vi "HexDAQ.vi"() -> ()   [LabVIEW 2016]
uses:
  input_params.ctl
  refs_front_panel.ctl
  <extravilib>/ChannelInstances/Tag-a[.](c(a[.](stamp),a[.](dbl)))/Read With Abort.vi
  <extravilib>/ChannelInstances/Tag-bool/Read With Abort.vi
  <extravilib>/ChannelInstances/Tag-t'Input_parameters.ctl'/Write With Abort.vi
  <extravilib>/ChannelInstances/Tag-str/Write With Abort.vi
  <extravilib>/ChannelInstances/Tag-bool/Write With Abort.vi
  <extravilib>/ChannelInstances/Tag-t'Input_parameters.ctl'/Instantiate.vi
  <extravilib>/ChannelInstances/Tag-str/Instantiate.vi
  <extravilib>/ChannelInstances/Tag-a[.](c(a[.](stamp),a[.](dbl)))/Instantiate.vi
  <extravilib>/ChannelInstances/Tag-t'Env_data.ctl'/Instantiate.vi
  <extravilib>/ChannelInstances/Tag-bool/Instantiate.vi
  <extravilib>/ChannelInstances/Tag-a[.](c(a[.](stamp),a[.](dbl)))/Endpoint.vi
  <extravilib>/ChannelInstances/Tag-bool/Endpoint.vi
  <extravilib>/ChannelInstances/Tag-t'Input_parameters.ctl'/Endpoint.vi
  <extravilib>/ChannelInstances/Tag-str/Endpoint.vi
  <extravilib>/ChannelInstances/Tag-bool.lvlib
  <extravilib>/ChannelInstances/Tag-a[.](c(a[.](stamp),a[.](dbl))).lvlib
  <extravilib>/ChannelInstances/Tag-str.lvlib
  <extravilib>/ChannelInstances/Tag-t'Input_parameters.ctl'.lvlib
  user32.dll
panel:
  in  "CV Switch Delay (s)":dbl
  in  "IV Switch Delay (s)":dbl
  in  "CV voltage file":path=path "C:/Users/Administrator/Desktop/HGCAL_sensor_tests/config/voltagesCV.txt"
  in  "IV voltage file":path=path "C:/Users/Administrator/Desktop/HGCAL_sensor_tests/config/voltagesIV.txt"
  in  "Abort 2":bool
  in  "Invert polarity":bool
  in  "No CV corrections":bool
  in  "Total curr/vlt \nevery x pads":i32=10
  in  "Disable Switchcard":bool
  in  "Comments (saved in data file)":string
  in  "Needle?":bool
  out "Total current":cluster{i32[], dbl[]}[](graph) caption="XY Graph"
  in  "CV voltage delay (s)":dbl=20.0
  in  "Sensor type":T1(ring)
  in  "Custom pad scan":string
  in  "Measurement type":T2(ring)=enum."Debug"
  in  "Hex pad numbers?":bool=TRUE
  in  "?":refnum<k7>(container)
  in  "Custom\nvoltages IV":string
  out "Single channel":cluster{"X array":dbl[], "Y array":dbl[]}[](graph) caption="XY Graph"
  in  "Repeat":i32=1
  in  "LCR signal voltage (V)":dbl=0.501
  in  "LCR signal frequenzy (kHz)":dbl=50.0 format="%#_13g"
  in  "Sampling number":i32=3
  in  "DMM device":T3(ring)=enum."Keithley6487"
  in  "Take environmental sensor data from":T4(ring)=enum."Switch Matrix"
  out "Environmental data":cluster{timestamp[], dbl[]}[](graph)
  out "Elapsed time":dbl format="%<%H:%M:%S>t"
  out "Estimated remaining time":dbl format="%<%H:%M:%S>t"
  out "Channel values":cluster{i32[], dbl[]}[](graph) caption="XY Graph"
  out "Current channel":dbl format="%#_13g"
  out "Current voltage (V)":dbl format="%#_13g"
  in  "Abort":bool
  in  "Output file":refnum<k7>(container) caption="Preview data file"
  in  "END DAQ":bool
  in  "START DAQ":bool
  in  "Custom\nvoltages CV":string
  in  "Data storage location (def: ./results)":path=path "C:/Users/Administrator/cernbox/HGCAL test results/Data"
  in  "Plot after execution?":bool=TRUE
  in  "Voltage limit (V)":dbl=1000.0
  in  "Compliance  level (uA)":dbl=500.0
  in  "VISA resource name LCR":refnum<visa-resource-name>="LCR_E4980"
  in  "VISA resource name DMM":refnum<visa-resource-name>="KEITHLEY_6487"
  in  "VISA resource name source":refnum<visa-resource-name>="Source_2410"
  in  "IV voltage delay (s)":dbl=5.0
  in  "Display/needle\nchannel":i32=144
  in  "Open after execution?":bool
  in  "Identifier (eg. wafer number)":string="Debug"
  # "HexDAQ\nThe LabVIEW program for HGCAL sensor tests\nFeedback and bug reports to andreas.alexander.maier@cern.ch"
  # "Measurement settings"
  # "Bookkeeping settings"
  # "VISA settings"
  # "Both are used to determine \nthe folder and file names"
  # "Device settings"
  # "Timing settings"
  # "Debug settings"
  # "Data processing settings"
  # "Ctrl+H for full display"
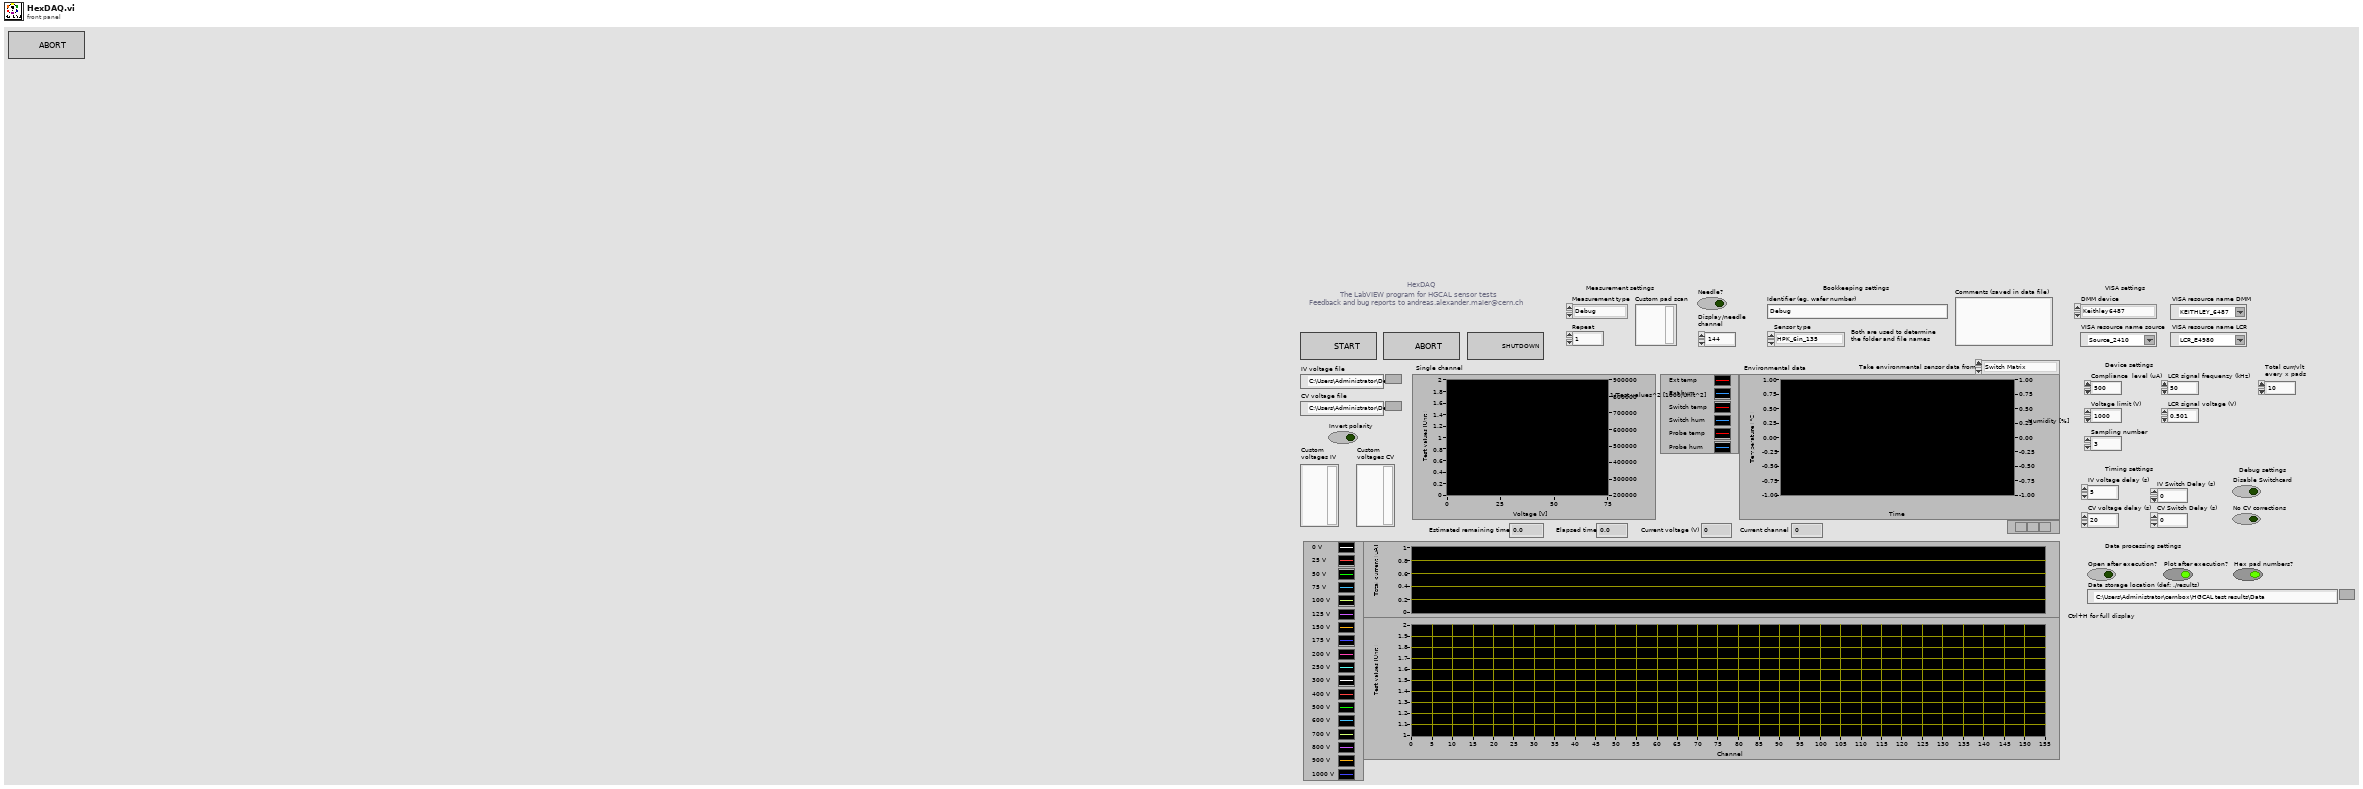
[diagram p1: front panel]
types:
  T1 = enum16{"HPK_6in_135", "HPK_8in_256", "IFX_8in_256", "Diode", "HPK_6in_256", "Full matrix"}
  T2 = enum16{"IV", "CV", "Debug", "Test_contact", "IV+CV"}
  T3 = enum16{"Keithley2001", "Keithley2450", "Keithley2410", "Keithley6487"}
  T4 = enum16{"Sensirion sht1x/7x", "Switch Matrix", "Probecard"}
  T5 = typedef "refs_front_panel.ctl" = cluster{"Current voltage (V)":refnum<vi>, "Elapsed time":refnum<vi>, "Current channel":refnum<vi>, "Abort":refnum<vi>, "Estimated remaining time":refnum<vi>, "Channel values XYGraph":refnum<vi>, "Single channel XYGraph":refnum<vi>, "Total current XYGraph":refnum<vi>}
  T6 = typedef "input_params.ctl" = cluster{"Measurement type":enum16{"IV", "CV", "Debug", "Test_contact"}, "Sensor type":enum16{"HPK_6in_135", "HPK_8in_256", "IFX_8in_256", "Diode", "HPK_6in_256", "Full matrix"}, "Identifier":string, "Open after execution?":bool, "Plot after execution?":bool, "Display channel":i32, "Voltage Delay (s)":dbl, "Switch Delay (s)":dbl, "VISA resource name source":refnum<visa-resource-name>, "VISA resource name DMM":refnum<visa-resource-name>, "VISA resource name LCR":refnum<visa-resource-name>, "Compliance  Level (A)":dbl, "Voltage Limit (V)":dbl, "Data storage location":string, "Scan voltages":string, "Use source as DMM?":bool, "LCR signal frequenzy (Hz)":dbl, "DMM device":enum16{"Keithley2001", "Keithley2450", "Keithley2410", "Keithley6487"}, "Sampling number":i32, "Use env. sensors on":enum16{"Sensirion sht1x/7x", "Switch Matrix", "Probecard"}, "Switchboard Handle":u32, "Use Switchboard":bool, "LCR signal voltage (V)":dbl, "Repeat":i32, "Scan voltages IV":string, "Scan voltages CV":string, "Hex pad numbers?":bool, "Set measurement type":enum16{"IV", "CV", "Debug", "Test_contact", "IV+CV"}, "Custom pad scan":string, "IV voltage Delay (s)":dbl, "CV voltage Delay (s)":dbl, "Needle measurement?":bool, "Comments":string, "LCR signal frequenzy (kHz)":dbl, "Compliance  Level (uA)":dbl, "Open Correction Array":dbl[][], "Current set voltage":dbl, "Last set voltage":dbl, "Current channel":i32, "Last OpenCorrection index":i32, "Total curr/vltg every x steps":i32, "Current channel iteration":i32, "No CV corrections":bool, "Mapfile":string, "Corrfile":string, "Invert polarity":bool, "IV voltage file":path, "CV voltage file":path, "IV Switch Delay (s)":dbl, "CV Switch Delay (s)":dbl}
  T7 = typedef "Tag-t'Input_parameters.ctl'.lvlib/))Channel.ctl" = refnum<queue>
  T8 = typedef "Tag-str.lvlib/))Channel.ctl" = refnum<queue>
  T9 = typedef "data_dynamic.ctl" = cluster{"Output file":path, "Y-label text":string, "Current set voltage":dbl, "Set voltage column":dbl[], "Pad number column":dbl[], "Data  column":dbl[], "Number of voltages":i32, "Compliance current (A)":dbl, "Geofile":string, "Peak voltage":dbl, "Hex PDF file":string, "Voltage array":dbl[], "Total current column":dbl[], "Timestamp column":dbl[], "Data name":string, "Data unit":string, "2nd data column":dbl[], "2nd data name":string, "2nd data unit":string, "3rd data column":dbl[], "4th data column":dbl[], "3rd data name":string, "3rd data unit":string, "4th data name":string, "4th data unit":string, "Actual voltage column":dbl[], "2nd Y-label text":string, "Single channel plot":path, "Temperature column":dbl[], "Humidity column":dbl[], "Channel switch array":i32[], "1st single plot name":string, "2nd single plot name":string, "All channels plot":path, "HexPlot command":string, "Custom channel array":i32[], "Data  error column":dbl[], "2nd data  error column":dbl[], "3rd data error column":dbl[], "4th data  error column":dbl[], "Total current plot":path, "5th data column":dbl[], "5th data  error column":dbl[], "6th data column":dbl[], "6th data  error column":dbl[], "5th data name":string, "5th data unit":string, "6th data name":string, "6th data unit":string, "HexPlot matrix command":string}
  T10 = typedef "Tag-bool.lvlib/))Channel.ctl" = refnum<queue>
  T11 = typedef "Tag-a[.](c(a[.](stamp),a[.](dbl))).lvlib/))Channel.ctl" = refnum<queue>
  T12 = typedef "Tag-t'Env_data.ctl'.lvlib/))Channel.ctl" = refnum<queue>
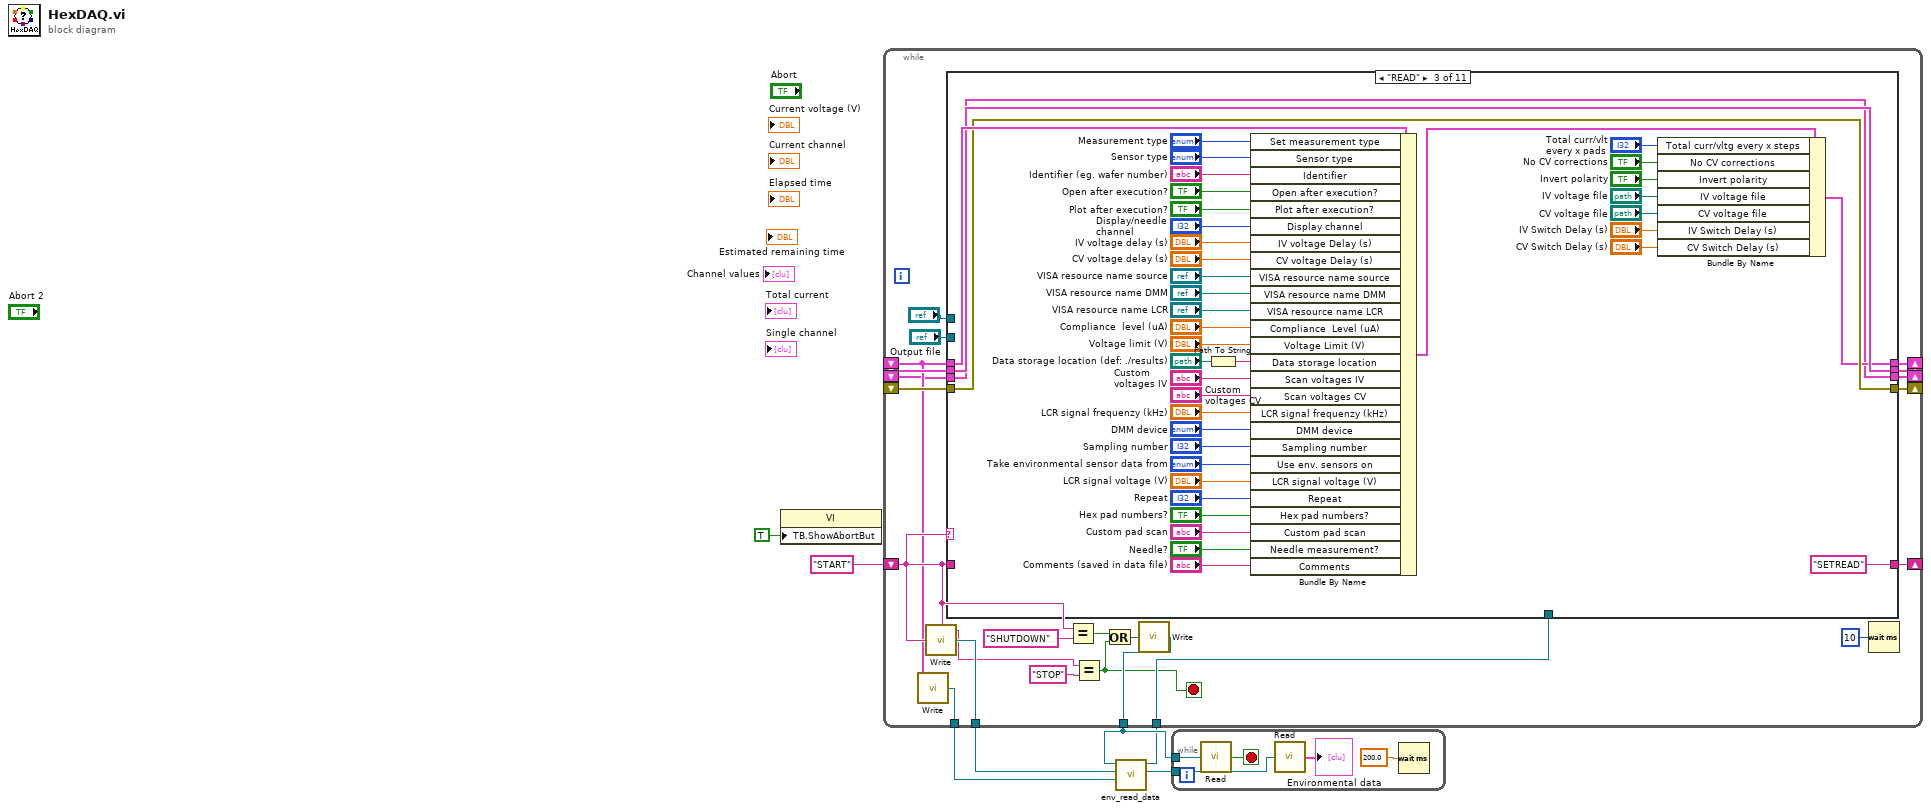
[diagram p0: block diagram]
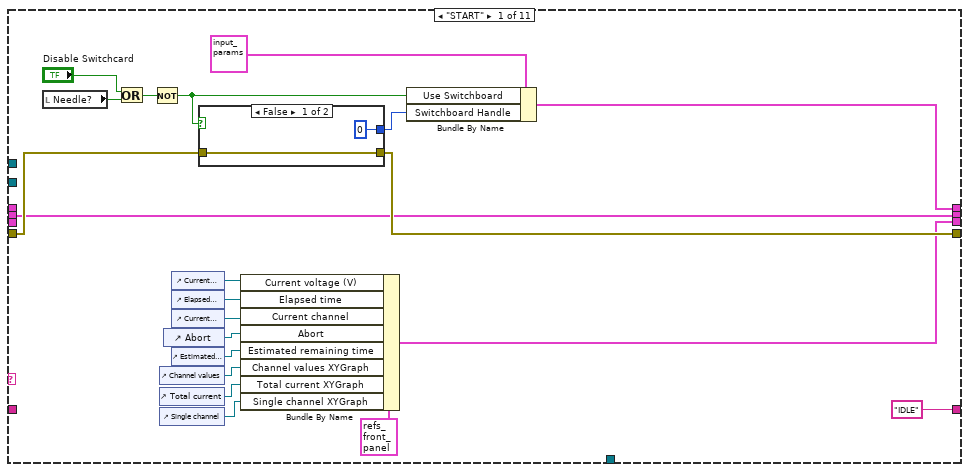
[diagram p2: hidden frame]
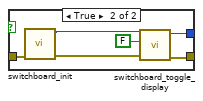
[diagram p3: hidden frame]
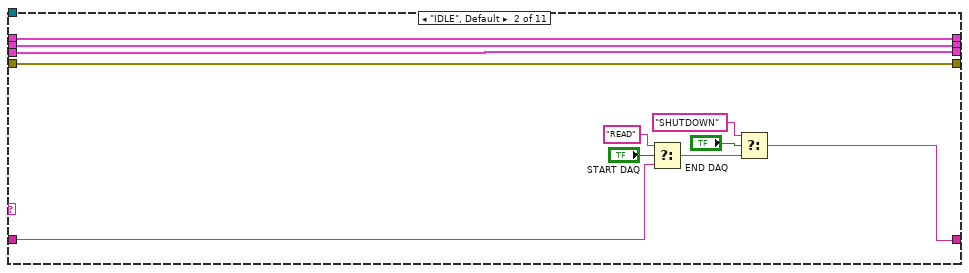
[diagram p4: hidden frame]
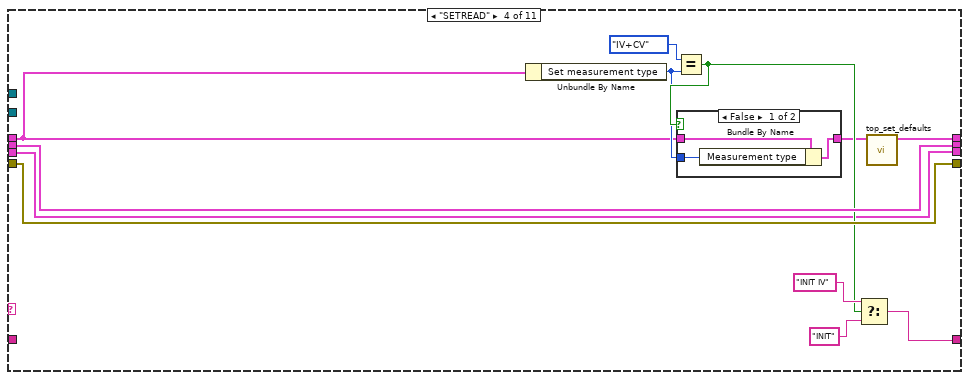
[diagram p5: hidden frame]
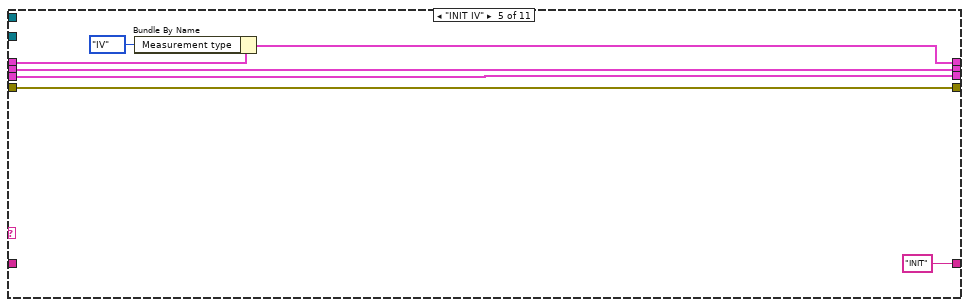
[diagram p7: hidden frame]
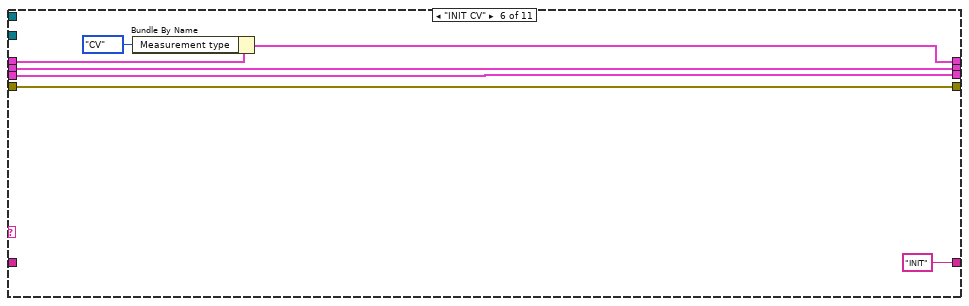
[diagram p8: hidden frame]
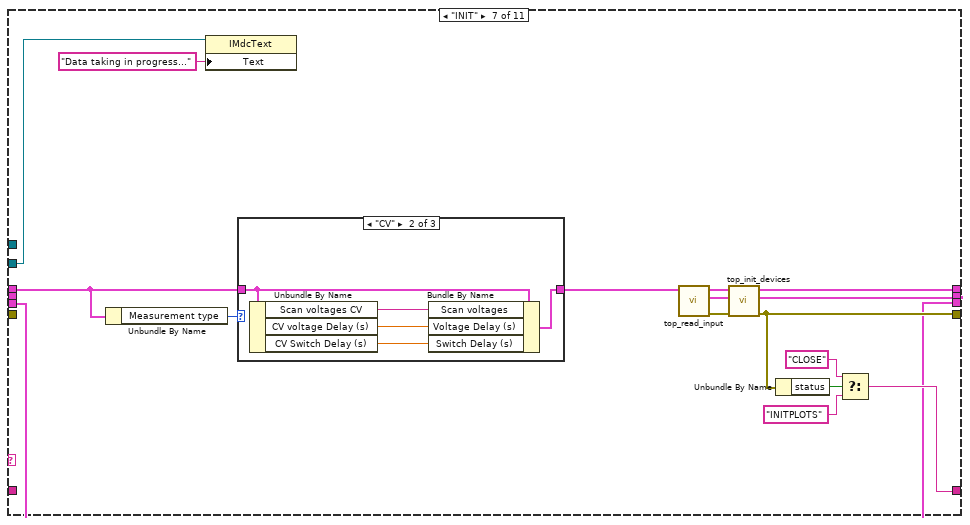
[diagram p9: hidden frame]
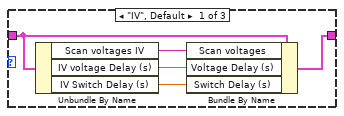
[diagram p10: hidden frame]
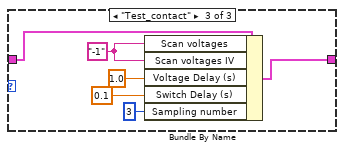
[diagram p11: hidden frame]
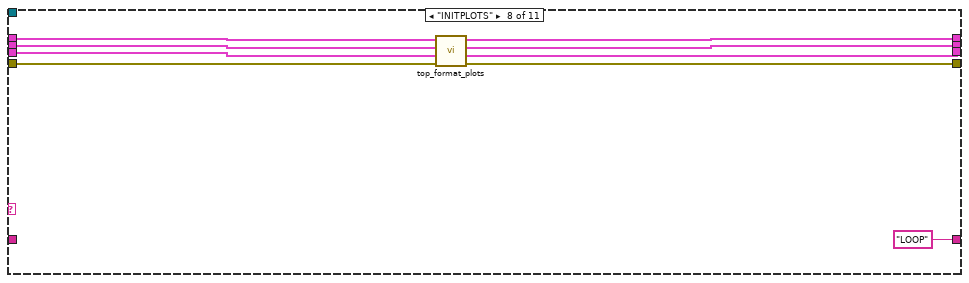
[diagram p12: hidden frame]
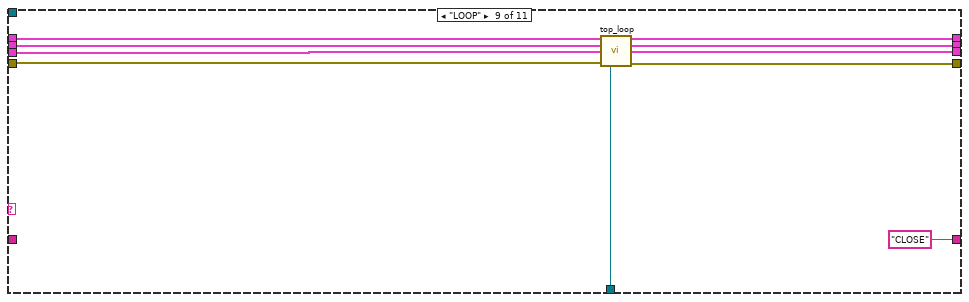
[diagram p13: hidden frame]
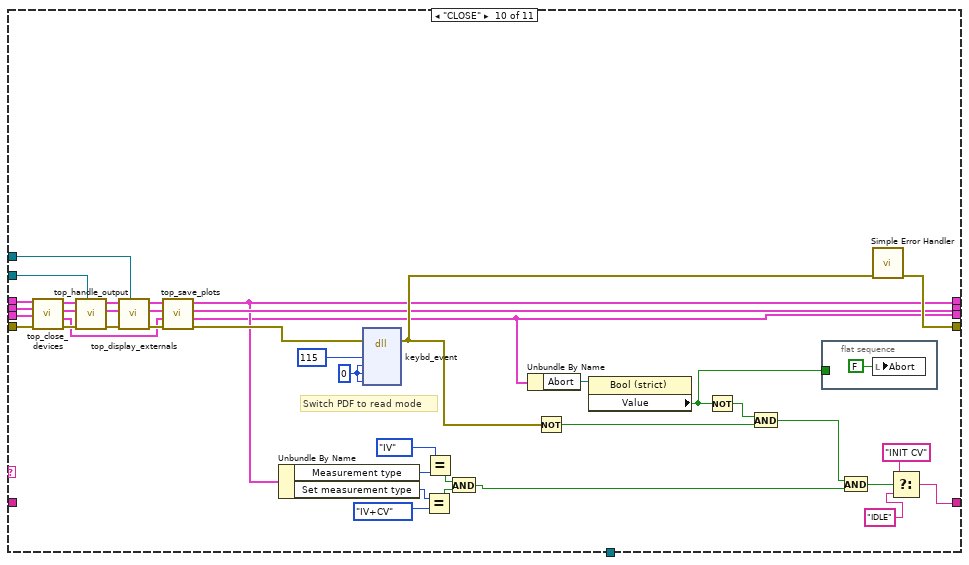
[diagram p14: hidden frame]
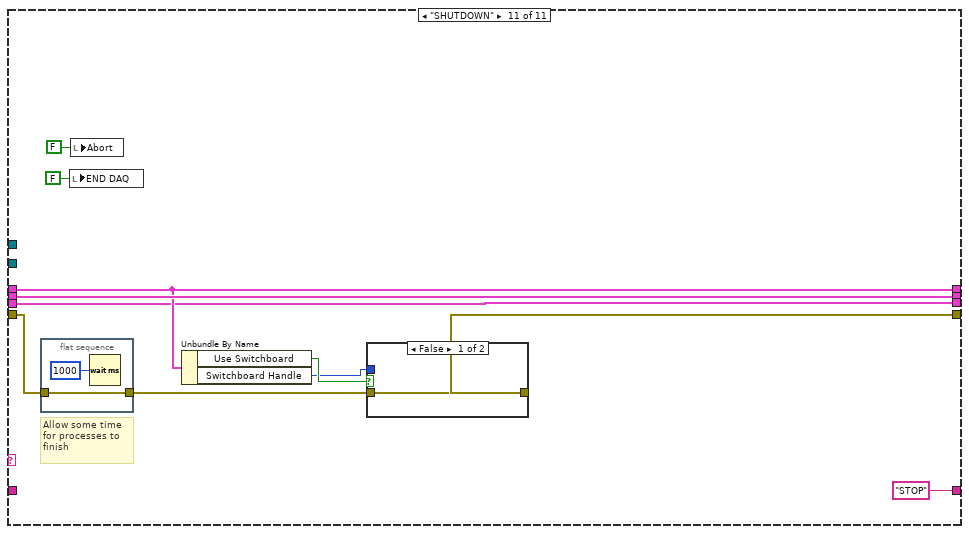
[diagram p15: hidden frame]
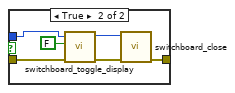
[diagram p16: hidden frame]
diagram:
  n1 = property class="VI"("TB.ShowAbortBut"=TRUE ("Tool Bar:Show Abort Button")) -> ()  [unwired: 2 in, 2 out]
  n2 = while {
    shift-right: [w29] -> _
    shift-left: "START" -> [w16]
    shift-right: [w24] -> _
    shift-left: _ -> [w22]
    shift-right: [w26] -> _
    shift-left: _ -> [w23]
    shift-right: [w25] -> _
    shift-left: _ -> [w11]
    tunnel: [w21] -> w5
    tunnel: w4 -> [w19]
    tunnel: [w18] -> w2
    tunnel: [w12] -> w1
    shift-right: [w9] -> _
    shift-left: _ -> [w8]
    stop <- w13 stop-if-true
    n3 = call <extravilib>:"Write.vi"("element"=w11) -> ("channel"=w12:T7)  [unwired: 1 out]
    n4 = call <extravilib>:"Write.vi"("element"=w16) -> ("channel"=w18:T8)  [unwired: 1 out]
    n5 = case shown="\"READ\"" w16 {
      tunnel: w16 -> [_ w69 _ _ _ _ _ _ _ _ _]
      tunnel: ["IDLE" ("t") w66 "SETREAD" ("t") w117 "INIT" ("t") "INIT" ("t") w145 "LOOP" ("t") "CLOSE" ("t") w210 "STOP" ("t")] -> w29
      tunnel: [w44 w62 w78 w113 w130 w137 w153 w177 w190 w200 w235] -> w25
      tunnel: [w48 w61 w88 w121 w133 w140 w149 w173 w188 w223 w239] -> w24
      tunnel: [w45 w60 w89 w122 w132 w139 w152 w176 w189 w202 w242] -> w26
      tunnel: w11 -> [_ w62 w90 w112 w131 w138 w142 w180 w185 w225 w235]
      tunnel: w23 -> [w45 w60 w89 w122 w132 w139 _ w181 w186 w220 w242]
      tunnel: w22 -> [w49 w61 w88 w121 w133 w140 _ w174 w187 w224 w237]
      tunnel: "Output file" -> [_ _ _ _ _ _ w150 _ _ w222 _]
      tunnel: "?" -> [_ _ _ _ _ _ _ _ _ w221 _]
      tunnel: w19 -> [_ _ _ _ _ _ _ _ w184 _ _]
      tunnel: [w30 w59 w75 w111 w127 w134 w141 w175 w183 w199 w234] -> w9
      tunnel: w8 -> [_ w59 w75 w111 w127 w134 w141 w178 w182 w193 w234]
      frame "START" {
        n6 = local read "Needle?"() -> (w41:bool)
        n7 = Or(x="Disable Switchcard", y=w41) -> (x .or. y?=w40:bool)
        n8 = Not(x=w40) -> (.not. x?=w43:bool)
        n9 = control-ref of="Channel values"() -> (w33:refnum<vi>)
        n10 = control-ref of="Total current"() -> (w32:refnum<vi>)
        n11 = control-ref of="Single channel"() -> (w31:refnum<vi>)
        n12 = control-ref of="Abort"() -> (w35:refnum<vi>)
        n13 = control-ref of="Current voltage (V)"() -> (w37:refnum<vi>)
        n14 = control-ref of="Elapsed time"() -> (w38:refnum<vi>)
        n15 = control-ref of="Current channel"() -> (w36:refnum<vi>)
        n16 = control-ref of="Estimated remaining time"() -> (w34:refnum<vi>)
        n17 = case shown="False" w43 {
          tunnel: w49 -> [w52 w58]
          tunnel: [w52 w57] -> w48
          tunnel: [u32 0 ("Handle") w55] -> w47
          frame False {
          }
          frame True {
            n18 = call <instrlib>:"switchboard_init.vi"("error in"=w58) -> ("error out"=w54:errorcluster, "Handle"=w53:u32)  [unwired: 9 in]
            n19 = call <instrlib>:"switchboard_toggle_display.vi"("error in"=w54, "On/Off"=FALSE, "Handle"=w53) -> ("error out"=w57:errorcluster, "Handle out"=w55:u32)  [unwired: 7 in]
          }
        }
        n20 = Bundle By Name(cluster=T5 {"Current voltage (V)"=refnum, "Elapsed time"=refnum, "Current channel"=refnum, "Abort"=refnum, "Estimated remaining time"=refnum, "Channel values XYGraph"=refnum, "Single channel XYGraph"=refnum, "Total current XYGraph"=refnum} ("Cluster"), "Current voltage (V)"=w37, "Elapsed time"=w38, "Current channel"=w36, "Abort"=w35, "Estimated remaining time"=w34, "Channel values XYGraph"=w33, "Total current XYGraph"=w32, "Single channel XYGraph"=w31) -> (w30:T5)
        n21 = Bundle By Name(cluster=T6 {"Measurement type"=enum."Debug", "Sensor type"=enum."HPK_6in_135", "Identifier"="test.txt", "Open after execution?"=FALSE, "Plot after execution?"=FALSE, "Display channel"=0, "Voltage Delay (s)"=0.5, "Switch Delay (s)"=0.01, "VISA resource name source"="", "VISA resource name DMM"="", "VISA resource name LCR"="", "Compliance  Level (A)"=10.0, "Voltage Limit (V)"=1000.0, "Data storage location"="", "Scan voltages"="", "Use source as DMM?"=FALSE, "LCR signal frequenzy (Hz)"=10.0, "DMM device"=enum."Keithley2001", "Sampling number"=1, "Use env. sensors on"=enum."Sensirion sht1x/7x", "Switchboard Handle"=0, "Use Switchboard"=FALSE, "LCR signal voltage (V)"=10000.0, "Repeat"=1, "Scan voltages IV"="", "Scan voltages CV"="", "Hex pad numbers?"=FALSE, "Set measurement type"=enum."Debug", "Custom pad scan"="", "IV voltage Delay (s)"=0.5, "CV voltage Delay (s)"=0.5, "Needle measurement?"=FALSE, "Comments"="test.txt", "LCR signal frequenzy (kHz)"=10.0, "Compliance  Level (uA)"=10.0, "Open Correction Array"=array2304x3[6912 elements], "Current set voltage"=0.0, "Last set voltage"=0.0, "Current channel"=0, "Last OpenCorrection index"=-1, "Total curr/vltg every x steps"=10, "Current channel iteration"=0, "No CV corrections"=FALSE, "Mapfile"="", "Corrfile"="", "Invert polarity"=FALSE, "IV voltage file"=path "", "CV voltage file"=path "", "IV Switch Delay (s)"=0.01, "CV Switch Delay (s)"=0.01} ("Input parameters 2"), "Use Switchboard"=w43, "Switchboard Handle"=w47) -> (w44:T6)
      }
      frame "IDLE", Default {
        n22 = Select(t="READ", s="START DAQ", f=w69) -> (s? t:f=w67:string)
        n23 = Select(t="SHUTDOWN", s="END DAQ", f=w67) -> (s? t:f=w66:string)
      }
      frame "READ" {
        n24 = Path To String(path="Data storage location (def: ./results)") -> (string=w93:string)
        n25 = Bundle By Name(cluster=w90, "Set measurement type"="Measurement type", "Sensor type"="Sensor type", "Identifier"="Identifier (eg. wafer number)", "Open after execution?"="Open after execution?", "Plot after execution?"="Plot after execution?", "Display channel"="Display/needle\nchannel", "IV voltage Delay (s)"="IV voltage delay (s)", "CV voltage Delay (s)"="CV voltage delay (s)", "VISA resource name source"="VISA resource name source", "VISA resource name DMM"="VISA resource name DMM", "VISA resource name LCR"="VISA resource name LCR", "Compliance  Level (uA)"="Compliance  level (uA)", "Voltage Limit (V)"="Voltage limit (V)", "Data storage location"=w93, "Scan voltages IV"="Custom\nvoltages IV", "Scan voltages CV"="Custom\nvoltages CV", "LCR signal frequenzy (kHz)"="LCR signal frequenzy (kHz)", "DMM device"="DMM device", "Sampling number"="Sampling number", "Use env. sensors on"="Take environmental sensor data from", "LCR signal voltage (V)"="LCR signal voltage (V)", "Repeat"="Repeat", "Hex pad numbers?"="Hex pad numbers?", "Custom pad scan"="Custom pad scan", "Needle measurement?"="Needle?", "Comments"="Comments (saved in data file)") -> (w79:T6)
        n26 = Bundle By Name(cluster=w79, "Total curr/vltg every x steps"="Total curr/vlt \nevery x pads", "No CV corrections"="No CV corrections", "Invert polarity"="Invert polarity", "IV voltage file"="IV voltage file", "CV voltage file"="CV voltage file", "IV Switch Delay (s)"="IV Switch Delay (s)", "CV Switch Delay (s)"="CV Switch Delay (s)") -> (w78:T6)
      }
      frame "SETREAD" {
        n27 = Unbundle By Name(w112) -> ("Set measurement type"=w115:T2)
        n28 = Equal?(x=T2."IV+CV" ("Measurement type"), y=w115) -> (x = y?=w116:bool)
        n29 = case shown="False" w116 {
          tunnel: w112 -> [w125 w126]
          tunnel: [w123 w126] -> w114
          tunnel: w115 -> [w124 _]
          frame False {
            n30 = Bundle By Name(cluster=w125, "Measurement type"=w124) -> (w123:T6)
          }
          frame True {
          }
        }
        n31 = Select(t="INIT IV", s=w116, f="INIT" ("t")) -> (s? t:f=w117:string)
        n32 = call "top_set_defaults.vi"("Input parameters"=w114) -> ("Input parameters out"=w113:T6)  [unwired: 10 in]
      }
      frame "INIT IV" {
        n33 = Bundle By Name(cluster=w131, "Measurement type"=enum16{"IV", "CV", "Debug", "Test_contact"}."IV") -> (w130:T6)
      }
      frame "INIT CV" {
        n34 = Bundle By Name(cluster=w138, "Measurement type"=enum16{"IV", "CV", "Debug", "Test_contact"}."CV") -> (w137:T6)
      }
      frame "INIT" {
        n35 = Unbundle By Name(w142) -> ("Measurement type"=w144:enum16{"IV", "CV", "Debug", "Test_contact"})
        n36 = property class="IMdcText"(reference=w150, "Text"="Data taking in progress...") -> ()  [unwired: 1 in, 2 out]
        n37 = case shown="\"CV\"" w144 {
          tunnel: w142 -> [w160 w165 w172]
          tunnel: [w159 w166 w171] -> w143
          frame "IV", Default {
            n38 = Unbundle By Name(w160) -> ("Scan voltages IV"=w161:string, "IV voltage Delay (s)"=w158:dbl, "IV Switch Delay (s)"=w157:dbl)
            n39 = Bundle By Name(cluster=w160, "Scan voltages"=w161, "Voltage Delay (s)"=w158, "Switch Delay (s)"=w157) -> (w159:T6)
          }
          frame "CV" {
            n40 = Unbundle By Name(w165) -> ("Scan voltages CV"=w164:string, "CV voltage Delay (s)"=w163:dbl, "CV Switch Delay (s)"=w162:dbl)
            n41 = Bundle By Name(cluster=w165, "Scan voltages"=w164, "Voltage Delay (s)"=w163, "Switch Delay (s)"=w162) -> (w166:T6)
          }
          frame "Test_contact" {
            w170 = "-1" ("Scan voltages")
            n42 = Bundle By Name(cluster=w172, "Scan voltages"=w170, "Scan voltages IV"=w170, "Voltage Delay (s)"=1.0, "Switch Delay (s)"=0.1, "Sampling number"=3) -> (w171:T6)
          }
        }
        n43 = call "top_read_input.vi"("Input parameters"=w143) -> ("error out"=w155:errorcluster, "Dynamic data"=w154:T9, "Input parameters"=w156:T6)  [unwired: 8 in]
        n44 = call "top_init_devices.vi"("error in (no error)"=w155, "Dynamic data"=w154, "Input parameters"=w156) -> ("error out"=w149:errorcluster, "Dynamic data"=w152:T9, "Input parameters"=w153:T6)  [unwired: 6 in]
        n45 = Unbundle By Name(w149) -> ("status"=w148:bool)
        n46 = Select(t="CLOSE", s=w148, f="INITPLOTS" ("t")) -> (s? t:f=w145:string)
      }
      frame "INITPLOTS" {
        n47 = call "top_format_plots.vi"("error in"=w174, "Front panel refs"=w178, "Dynamic data"=w181, "Input parameters"=w180) -> ("error out"=w173:errorcluster, "Front panel refs out"=w175:T5, "Dynamic data out"=w176:T9, "Input parameters out"=w177:T6)  [unwired: 4 in]
      }
      frame "LOOP" {
        n48 = call "top_loop.vi"("Input parameters"=w185, "Dynamic data"=w186, "Front_panel_refs"=w182, "error in (no error)"=w187, "Environmental data"=w184) -> ("Input parameters out"=w190:T6, "Dynamic data out"=w189:T9, "Front_panel_refs out"=w183:T5, "error out"=w188:errorcluster)  [unwired: 7 in]
      }
      frame "CLOSE" {
        w207 = u8 0 ("bScan")
        # "Switch PDF to read mode"
        n49 = call "top_close_devices.vi"("error in (no error)"=w224, "Front_panel_refs"=w193, "Dynamic data"=w220, "Input parameters"=w225) -> ("error out"=w231:errorcluster, "Front_panel_refs out"=w192:T5, "Dynamic data"=w229:T9, "Input parameters"=w230:T6)  [unwired: 4 in]
        n50 = call "top_handle_output.vi"("Output file text box"=w222, "error in (no error)"=w231, "Dynamic data"=w229, "Input parameters"=w230) -> ("error out"=w228:errorcluster, "Dynamic data"=w227:T9, "Input parameters"=w226:T6)  [unwired: 5 in]
        n51 = call "top_display_externals.vi"("AcroPDF"=w221, "error in (no error)"=w228, "Dynamic data"=w227, "Input parameters"=w226) -> ("error out"=w219:errorcluster, "Dynamic data"=w203:T9, "Input parameters"=w201:T6)  [unwired: 5 in]
        n52 = call "top_save_plots.vi"("error in"=w219, "Front_panel_refs"=w192, "Dynamic data"=w203, "Input parameters"=w201) -> ("error out"=w205:errorcluster, "Front_panel_refs out"=w199:T5, "Dynamic data out"=w202:T9, "Input parameters out"=w200:T6)  [unwired: 4 in]
        n53 = Unbundle By Name(w200) -> ("Measurement type"=w218:enum16{"IV", "CV", "Debug", "Test_contact"}, "Set measurement type"=w216:T2)
        n54 = dll-call lib="user32.dll" fn="keybd_event"(error in=w205, "bVk"=u8 115 ("Virtual Key"), "bScan"=w207, "dwFlags"=w207, "dwExtraInfo"=w207) -> (error out=w204:errorcluster)  [unwired: 7 in, 1 out]
        n55 = Equal?(x=w216, y=T2."IV+CV") -> (x = y?=w213:bool)
        n56 = Equal?(x=enum16{"IV", "CV", "Debug", "Test_contact"}."IV", y=w218) -> (x = y?=w214:bool)
        n57 = And(x=w214, y=w213) -> (x .and. y?=w195:bool)
        n58 = Unbundle By Name(w199) -> ("Abort"=w198:refnum<vi>)
        n59 = Not(x=w204) -> (.not. x?=w196:bool)
        n60 = property class="Bool (strict)"(reference=w198) -> ("Value"=w209:bool)  [unwired: 1 in, 2 out]
        n61 = Not(x=w209) -> (.not. x?=w197:bool)
        n62 = And(x=w197, y=w196) -> (x .and. y?=w194:bool)
        n63 = flat-sequence {
          tunnel: w209 -> [_]
          frame #0 {
            n64 = local write "Abort"(FALSE ("Abort")) -> ()
          }
        }
        n65 = And(x=w194, y=w195) -> (x .and. y?=w208:bool)
        n66 = call <vilib>:"Simple Error Handler.vi"("error in (no error)"=w204) -> ("error out"=w223:errorcluster)  [unwired: 4 in, 4 out]
        n67 = Select(t="INIT CV", s=w208, f="IDLE" ("t")) -> (s? t:f=w210:string)
      }
      frame "SHUTDOWN" {
        # "Allow some time\nfor processes to\nfinish"
        n68 = flat-sequence {
          tunnel: w237 -> [w244]
          tunnel: [w244] -> w236
          frame #0 {
            n69 = Wait (ms)(milliseconds to wait=u32 1000) -> ()  [unwired: 1 out]
          }
        }
        n70 = local write "END DAQ"(FALSE ("END DAQ")) -> ()
        n71 = local write "Abort"(FALSE ("Abort")) -> ()
        n72 = Unbundle By Name(w235) -> ("Use Switchboard"=w241:bool, "Switchboard Handle"=w240:u32)
        n73 = case shown="False" w241 {
          tunnel: w236 -> [w246 w250]
          tunnel: [w246 w252] -> w239
          tunnel: w240 -> [_ w249]
          frame False {
          }
          frame True {
            n74 = call <instrlib>:"switchboard_toggle_display.vi"("error in"=w250, "On/Off"=FALSE, "Handle"=w249) -> ("error out"=w247:errorcluster, "Handle out"=w248:u32)  [unwired: 7 in]
            n75 = call <instrlib>:"switchboard_close.vi"("error in"=w247, "Handle"=w248) -> ("error out"=w252:errorcluster)  [unwired: 8 in, 1 out]
          }
        }
      }
    }
    n76 = Equal?(x=w16, y="SHUTDOWN") -> (x = y?=w15:bool)
    n77 = Equal?(x=w16, y="STOP") -> (x = y?=w13:bool)
    n78 = Or(x=w15, y=w13) -> (x .or. y?=w14:bool)
    n79 = call <extravilib>:"Write.vi"("element"=w14) -> ("channel"=w21:T10)  [unwired: 1 out]
    n80 = Wait (ms)(milliseconds to wait=u32 10) -> ()  [unwired: 1 out]
  }
  n81 = call "env_read_data.vi"("Input parameters"=w1, "State"=w2, "Stop signal"=w5) -> ("Plot data out"=w3:T11, "Env data out"=w4:T12)  [unwired: 6 in, 1 out]
  n82 = while {
    tunnel: w5 -> [w255]
    tunnel: w3 -> [w253]
    stop <- w254 stop-if-true
    n83 = call <extravilib>:"Read.vi"("channel"=w255) -> ("element"=w254:bool)  [unwired: 1 in, 1 out]
    n84 = call <extravilib>:"Read.vi"("channel"=w253) -> ("element"=→"Environmental data":cluster{timestamp[], dbl[]}[])  [unwired: 1 in, 1 out]
    n85 = Wait (ms)(milliseconds to wait=sgl 200.0 ("Sample period (s)")) -> ()  [unwired: 1 out]
  }
